vi "Sub_SPCI_str_to_data.vi"(1 "Convert To":enum16{".csv", ".xlsx", ".txt"}(ring), 2 "SCPI In":T1) -> (0 "Data Out":cluster{"Time/s":dbl[][], "Current/A":dbl[][]})   [LabVIEW 2014]
uses:
  dll/Save2Darr_to_csv.dll
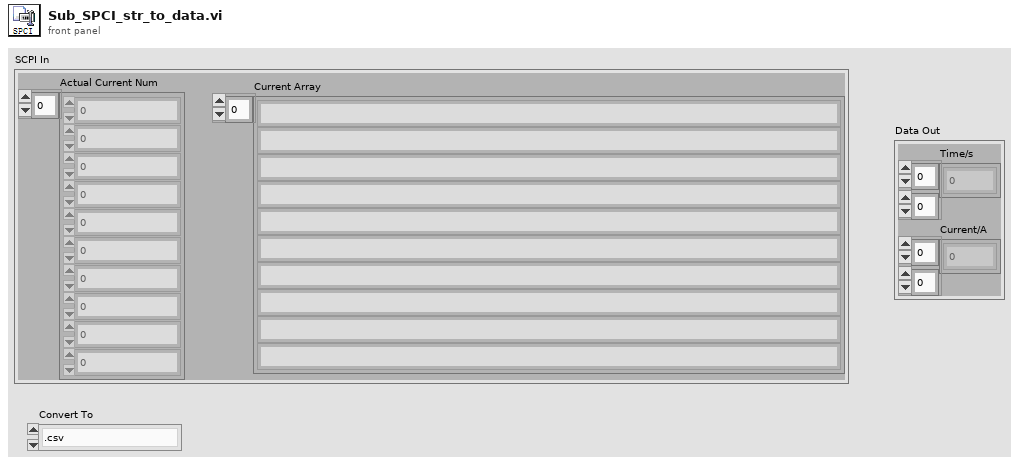
[diagram p1: front panel]
types:
  T1 = cluster{"Current Array":string[], "Actual Current Num":i32[]}
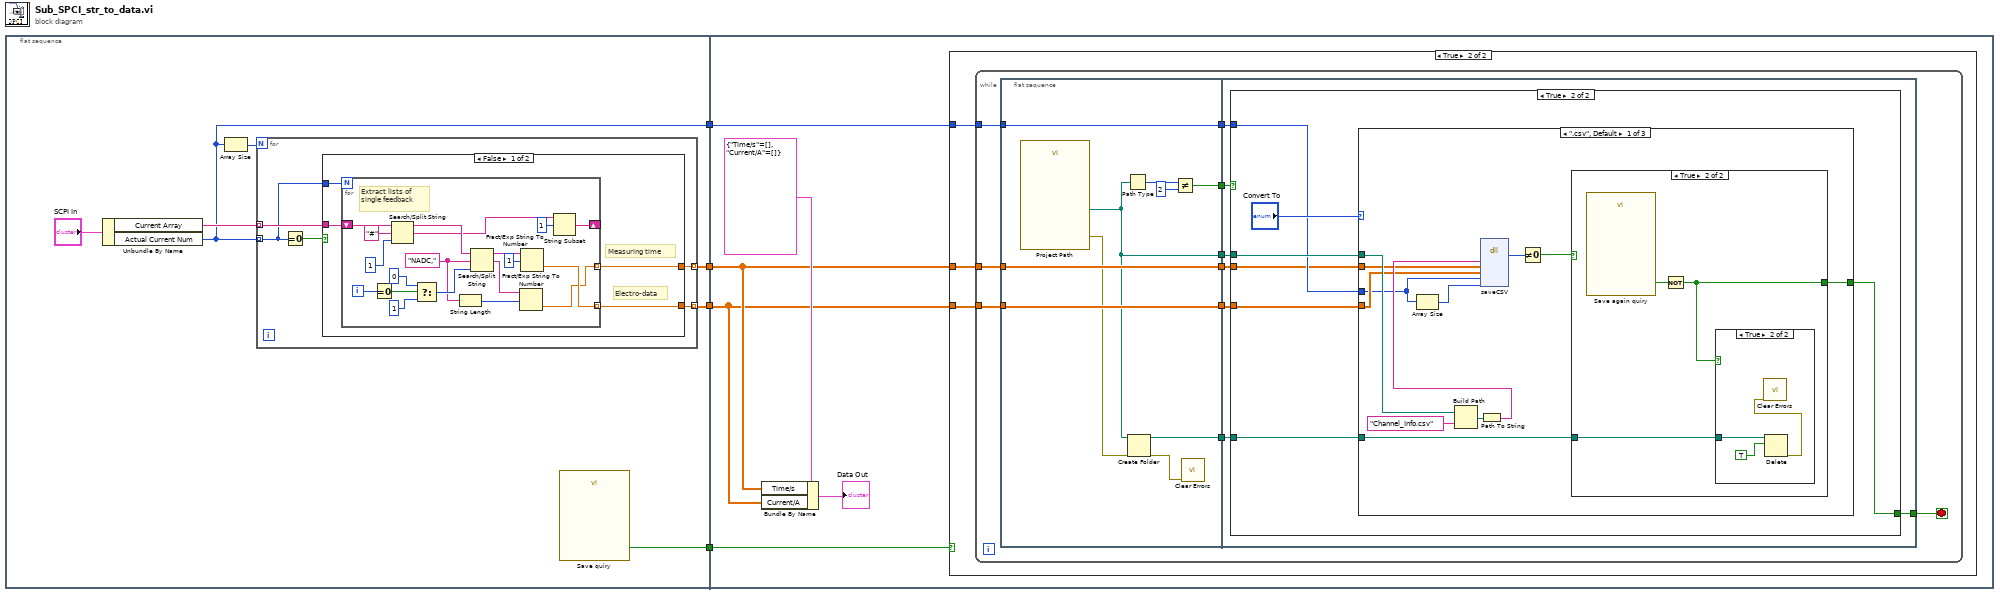
[diagram p0: block diagram]
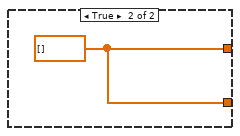
[diagram p2: hidden frame]
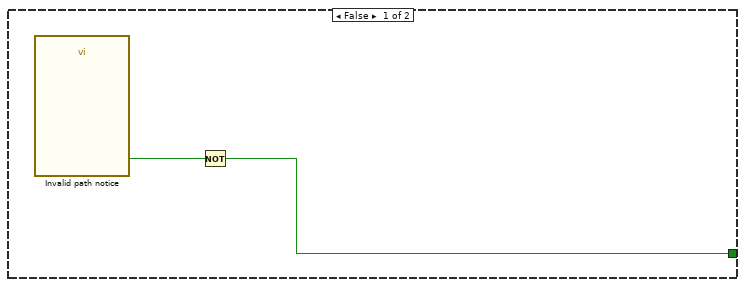
[diagram p4: hidden frame]
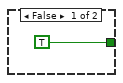
[diagram p5: hidden frame]
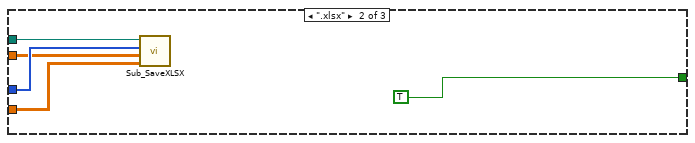
[diagram p7: hidden frame]
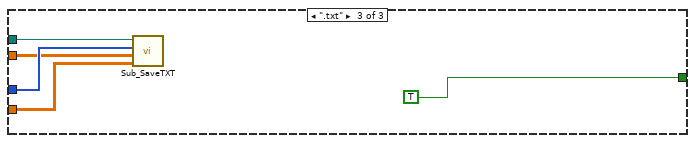
[diagram p8: hidden frame]
diagram:
  n1 = flat-sequence {
    tunnel: [w8] -> w4
    tunnel: [w7] -> w3
    tunnel: [w6] -> w2
    tunnel: [w5] -> w1
    tunnel: w4 -> [w43]
    tunnel: w3 -> [w42]
    tunnel: w2 -> [w46]
    tunnel: w1 -> [w45]
    frame #0 {
      n2 = Unbundle By Name("SCPI In") -> ("Current Array"=w9:string[], "Actual Current Num"=w6:i32[])
      n3 = Array Size(array=w6) -> (size(s)=w10:i32)
      n4 = for {
        N: w10 -> [_]
        tunnel: w6 -> [w14] mode=indexing
        tunnel: w9 -> [w15] mode=indexing
        tunnel: [w13] -> w8 mode=indexing
        tunnel: [w12] -> w7 mode=indexing
        n5 = Equal To 0?(x=w14) -> (x = 0?=w16:bool)
        n6 = case shown="False" w16 {
          tunnel: w15 -> [w20 _]
          tunnel: w14 -> [w19 _]
          tunnel: [w18 w40] -> w13
          tunnel: [w17 w40] -> w12
          frame False {
            # "Measuring time"
            # "Electro-data"
            n7 = for {
              N: w19 -> [_]
              shift-right: [w23] -> _
              shift-left: w20 -> [w38]
              tunnel: [w24] -> w18 mode=indexing
              tunnel: [w25] -> w17 mode=indexing
              i -> [w35]
              w29 = "NADC," ("search string/char (-)")
              # "Extract lists of \nsingle feedback"
              n8 = Equal To 0?(x=w35) -> (x = 0?=w34:bool)
              n9 = Search/Split String(string=w38, search string/char (-)="#", offset (0)=1) -> (substring before match=w36:string, match + rest of string=w22:string)  [unwired: 1 out]
              n10 = Select(t=0 ("offset (0)"), s=w34, f=1 ("offset (0)")) -> (s? t:f=w31:i32)
              n11 = String Length(string=w29) -> (length=w27:i32)
              n12 = Search/Split String(string=w36, search string/char (-)=w29, offset (0)=w31) -> (substring before match=w30:string, match + rest of string=w28:string)  [unwired: 1 out]
              n13 = Fract/Exp String To Number(string=w28, offset=w27) -> (number=w24:dbl)  [unwired: 2 in, 1 out]
              n14 = Fract/Exp String To Number(string=w30, offset=1) -> (number=w25:dbl)  [unwired: 2 in, 1 out]
              n15 = String Subset(string=w22, offset (0)=1) -> (substring=w23:string)  [unwired: 1 in]
            }
          }
          frame True {
            w40 = dbl[] []
          }
        }
      }
      n16 = call "Save quiry"() -> ("OK"=w5:bool)  [unwired: 10 in, 1 out]
    }
    frame #1 {
      n17 = Bundle By Name(cluster=cluster{"Time/s":dbl[][], "Current/A":dbl[][]} {"Time/s"=[], "Current/A"=[]}, "Time/s"=w43, "Current/A"=w42) -> (→"Data Out":cluster{"Time/s":dbl[][], "Current/A":dbl[][]})
      n18 = case shown="True" w45 {
        tunnel: w46 -> [_ w49]
        tunnel: w43 -> [_ w48]
        tunnel: w42 -> [_ w47]
        frame False {
        }
        frame True {
          n19 = while {
            tunnel: w49 -> [w58]
            tunnel: w48 -> [w53]
            tunnel: w47 -> [w51]
            stop <- w57 stop-if-true
            n20 = flat-sequence {
              tunnel: [w67] -> w59
              tunnel: w58 -> [w66]
              tunnel: [w66] -> w56
              tunnel: [w63] -> w55
              tunnel: [w65] -> w54
              tunnel: w53 -> [w65]
              tunnel: [w64] -> w52
              tunnel: w51 -> [w64]
              tunnel: [w62] -> w50
              tunnel: w59 -> [w76]
              tunnel: [w75] -> w57
              tunnel: w56 -> [w74]
              tunnel: w55 -> [w73]
              tunnel: w54 -> [w72]
              tunnel: w52 -> [w71]
              tunnel: w50 -> [w70]
              frame #0 {
                n21 = call "Project Path"() -> ("selected path"=w63:path, "error out"=w60:errorcluster)  [unwired: 12 in, 2 out]
                n22 = Path Type(1:w63) -> (0:w69:i16)
                n23 = Create Folder(path (use dialog)=w63, error in=w60) -> (created path=w62:path, error out=w61:errorcluster)  [unwired: 1 in, 1 out]
                n24 = Not Equal?(x=w69, y=i16 2) -> (x != y?=w67:bool)
                n25 = call <vilib>:"Clear Errors.vi"("error in (no error)"=w61) -> ()  [unwired: 5 in, 2 out]
              }
              frame #1 {
                n26 = case shown="True" w76 {
                  tunnel: [w77 w80] -> w75
                  tunnel: w74 -> [_ w83]
                  tunnel: w73 -> [_ w84]
                  tunnel: w72 -> [_ w82]
                  tunnel: w71 -> [_ w81]
                  tunnel: w70 -> [_ w79]
                  frame False {
                    n27 = call "Invalid path notice"() -> ("OK"=w78:bool)  [unwired: 10 in, 1 out]
                    n28 = Not(x=w78) -> (.not. x?=w77:bool)
                  }
                  frame True {
                    n29 = case shown="\".csv\", Default" "Convert To" {
                      tunnel: w84 -> [w96 w109 w114]
                      tunnel: w83 -> [w90 w108 w113]
                      tunnel: w82 -> [w93 w107 w112]
                      tunnel: w81 -> [w92 w106 w111]
                      tunnel: [w88 TRUE TRUE] -> w80
                      tunnel: w79 -> [w87 _ _]
                      frame ".csv", Default {
                        n30 = Array Size(array=w90) -> (size(s)=w91:i32)
                        n31 = Build Path(base path=w96, name or relative path="Channel_Info.csv") -> (appended path=w95:path)
                        n32 = Path To String(path=w95) -> (string=w94:string)
                        n33 = dll-call lib="C:/Users/DrippySummer/Documents/LabVIEW Data/SavaData/MultiChannelKeithley/dll/Save2Darr_to_csv.dll" fn="saveCSV"("FileName"=w94, "x_2D_arr"=w93, "y_2D_arr"=w92, "validity_arr"=w90, "validity_len"=w91) -> ("State"=w89:i32)  [unwired: 8 in, 2 out]
                        n34 = Not Equal To 0?(x=w89) -> (x != 0?=w86:bool)
                        n35 = case shown="True" w86 {
                          tunnel: [TRUE w100] -> w88
                          tunnel: w87 -> [_ w99]
                          frame False {
                          }
                          frame True {
                            n36 = call "Save again quiry"() -> ("OK"=w101:bool)  [unwired: 10 in, 1 out]
                            n37 = Not(x=w101) -> (.not. x?=w100:bool)
                            n38 = case shown="True" w100 {
                              tunnel: w99 -> [_ w103]
                              frame False {
                              }
                              frame True {
                                n39 = Delete(path (use dialog)=w103, entire hierarchy (F)=TRUE) -> (error out=w102:errorcluster)  [unwired: 3 in, 2 out]
                                n40 = call <vilib>:"Clear Errors.vi"("error in (no error)"=w102) -> ()  [unwired: 5 in, 2 out]
                              }
                            }
                          }
                        }
                      }
                      frame ".xlsx" {
                        n41 = call "Sub_SaveXLSX.vi"("y_var"=w106, "x_var"=w107, "Validity"=w108, "DirPath"=w109) -> ()
                      }
                      frame ".txt" {
                        n42 = call "Sub_SaveTXT.vi"("y_var"=w111, "x_var"=w112, "Validity"=w113, "DirPath"=w114) -> ()
                      }
                    }
                  }
                }
              }
            }
          }
        }
      }
    }
  }
